vi "GeneratorConfigure.vi"(0 "VISA resource name":refnum<visa-resource-name>, 1 "Amplitude Unit (0: Vpp)":i32(ring) items=["Vpp", "Vrms", "dBm"], 2 "Amplitude (5 Vpp)":dbl=3.3, 3 "Offset (0)":dbl=1.65, 5 "Output Channel (1: Channel 1)":i32(ring)=1 items=["Channel 1"=1, "Channel 2"=2], 7 "Enable Output (T: Enable)":bool=TRUE, 9 "Enable Align (F: Disable)":bool, 11 "error in (no error)":errorcluster, 12 "Frequency (1000 Hz)":dbl=20.0, 13 "Duty Cycle (50 %)":dbl=20.0, 14 "Phase (0 Degree)":dbl) -> (4 "VISA resource name out":refnum<visa-resource-name>, 15 "error out":errorcluster)   [LabVIEW 2018]
panel:
  out "output string":string
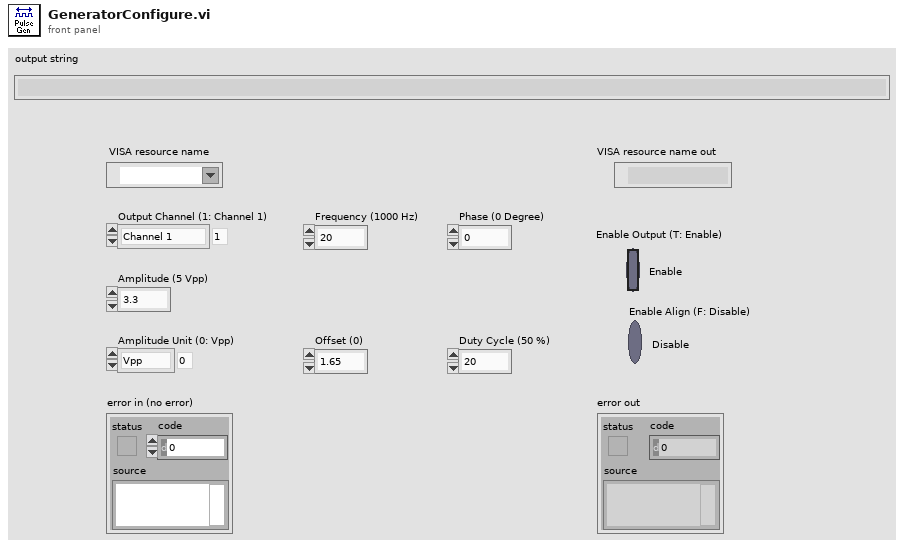
[diagram p1: front panel]
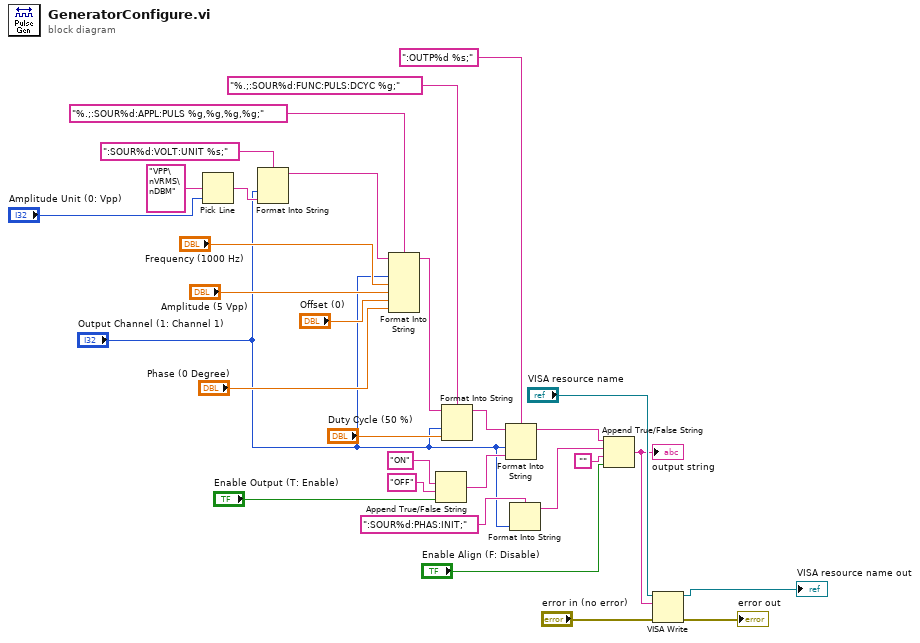
[diagram p0: block diagram]
diagram:
  n1 = Pick Line(multi-line string="VPP\nVRMS\nDBM", line index="Amplitude Unit (0: Vpp)") -> (output string=w19:string)  [unwired: 1 out]
  n2 = Format Into String(format string=":SOUR%d:VOLT:UNIT %s;", "Output Channel (1: Channel 1)", w19) -> (resulting string=w16:string)  [unwired: 2 in, 1 out]
  n3 = Format Into String(format string="%.;:SOUR%d:APPL:PULS %g,%g,%g,%g;", initial string=w16, "Output Channel (1: Channel 1)", "Frequency (1000 Hz)", "Amplitude (5 Vpp)", "Offset (0)", "Phase (0 Degree)") -> (resulting string=w25:string)  [unwired: 1 in, 1 out]
  n4 = Append True/False String(1:"Enable Output (T: Enable)", 2:"OFF", 3:"ON") -> (0:w11:string)  [unwired: 1 out]
  n5 = Format Into String(format string="%.;:SOUR%d:FUNC:PULS:DCYC %g;", initial string=w25, "Output Channel (1: Channel 1)", "Duty Cycle (50 %)") -> (resulting string=w10:string)  [unwired: 1 in, 1 out]
  n6 = Format Into String(format string=":OUTP%d %s;", initial string=w10, "Output Channel (1: Channel 1)", w11) -> (resulting string=w3:string)  [unwired: 1 in, 1 out]
  n7 = Format Into String(format string=":SOUR%d:PHAS:INIT;", "Output Channel (1: Channel 1)") -> (resulting string=w4:string)  [unwired: 2 in, 1 out]
  n8 = Append True/False String(1:"Enable Align (F: Disable)", 2:"", 3:w4, 4:w3) -> (0:w6:string)
  "output string" <- w6
  n9 = VISA Write(VISA resource name="VISA resource name", write buffer=w6, error in (no error)="error in (no error)") -> (VISA resource name out=→"VISA resource name out":refnum<visa-resource-name>, error out=→"error out":errorcluster)  [unwired: 1 out]
